vi "Test JSON Config.vi"() -> ()   [LabVIEW 2021]
uses:
  Source/Abs_Types/Double Float/Support/Type.ctl
  Source/Abs_Types/Boolean_1D/Support/Element Type.ctl
  Source/Constants/Support/DBL_1D/Type.ctl
  Source/Abs_Types/Double Float 1D/Support/Type.ctl
  Source/Abs_Types/Boolean/Abs_Boolean.lvclass
  C:/New folder/LV_Abstract/LV_Abstract/Source/Abs_Types/Type/Abs_Type.lvclass
  Source/Constants/Support/Bool_1D/Const_Bool_1D.lvclass
  Source/Abs_Types/Boolean_1D/Abs_Boolean_1D.lvclass
  Source/Constants/Support/DBL_1D/Const_DBL_1D.lvclass
  Source/Abs_Types/Type/Abs_Type.lvclass
  Source/Abs_Types/Double Float 1D/Abs_Double Float 1D.lvclass
  Source/Constants/Support/Bool_1D/Const_Bool_1D.lvclass/Const_Bool_1D.ctl
  Source/Constants/Support/DBL_1D/Const_DBL_1D.lvclass/Const_DBL_1D.ctl
  Source/Abs_Types/Type/Abs_Type.lvclass/Abs_Type.ctl
  Source/Abs_Types/Double Float/Abs_Double Float.lvclass
  Source/Abs_Types/String/Abs_String.lvclass
  Source/Abs_Types/String/Simple Read.vi
  Source/Abs_Types/Boolean/Simple Read.vi
  Source/Abs_Types/Double Float/Simple Read.vi
  Source/Constants/Support/DBL_1D/Properties/Write Value.vi
  Source/Constants/Support/Bool_1D/Properties/Write Value.vi
  Source/Abs_Types/Type/Properties/Write Name.vi
  Source/Abs_Types/Type/Properties/Read Name.vi
  Source/Constants/Support/Bool/Bool.vi
  Source/Functions/Logic/Support/OR/Bool/Method.vi
  Source/Constants/Support/DBL/DBL.vi
  Source/Constants/Support/Str/Str.vi
  Source/Constants/Support/DBL/Const_DBL.lvclass
  Source/Constants/Support/Bool/Const_Bool.lvclass
  Source/Functions/Logic/Support/OR/Bool/OR_Bool.lvclass
  Source/Constants/Support/Str/Const_Str.lvclass
panel:
  out "Value 3":T1
  out "JSON 6":string
  in  "Value 2":T2
  out "Boolean 1D":T3[](array[typedef])
  out "JSON":string
  in  "Array Value":bool[](array[boolean])
  out "Name":string
  out "JSON 5":string
  out "Boolean 6":bool
  in  "Boolean 5":bool
  in  "Boolean 4":bool
  out "String 2":string
  out "JSON 4":string
  in  "String":string
  out "Value":T4
  out "JSON 3":string
  in  "Numeric":dbl
  in  "Boolean 2":bool
  out "Boolean":bool
  out "JSON 2":string
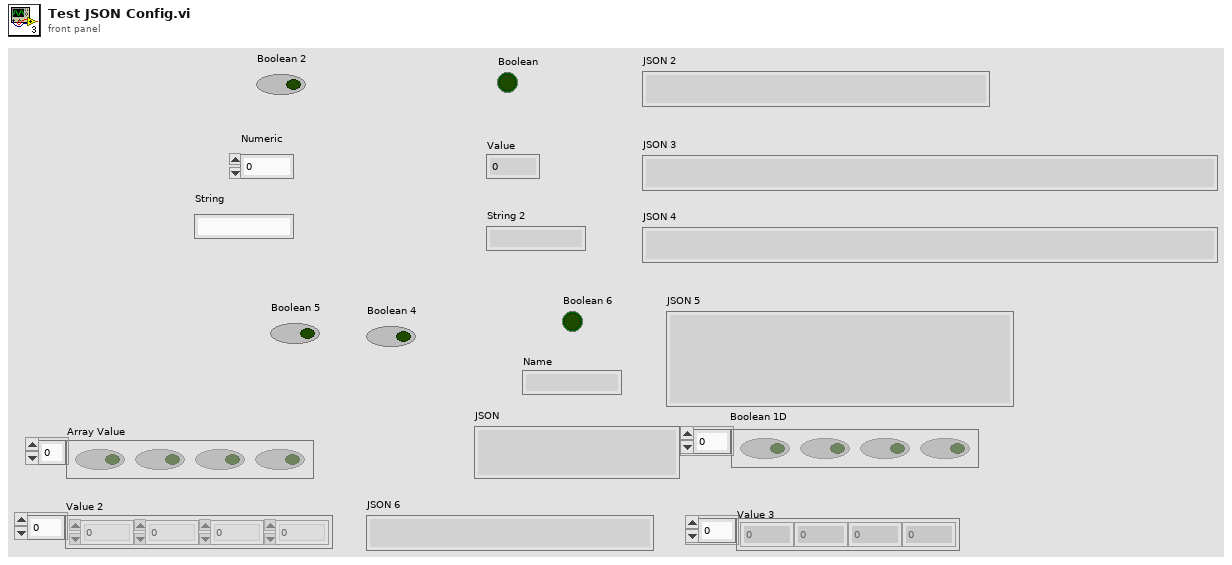
[diagram p1: front panel]
types:
  T1 = typedef "Abs_Double Float 1D.lvclass/Type.ctl" = dbl[]
  T2 = typedef "Const_DBL_1D.lvclass/Type.ctl" = dbl[]
  T3 = typedef "Abs_Boolean_1D.lvclass/Element Type.ctl" = bool
  T4 = typedef "Abs_Double Float.lvclass/Type.ctl" = dbl
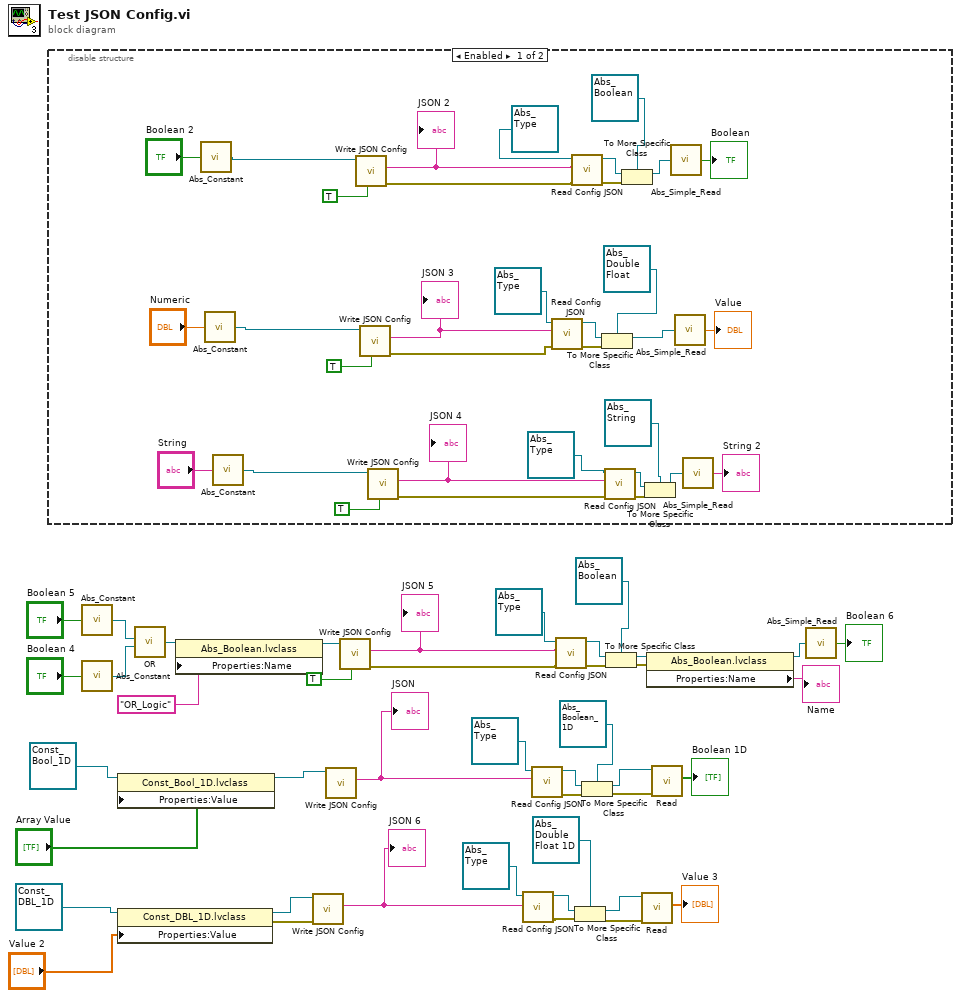
[diagram p0: block diagram]
diagram:
  n1 = disable-structure shown="Enabled" {
    frame Enabled {
      n2 = call-poly "Abs_Constant.vi"("Boolean"="Boolean 2") -> ("Abs_Boolean.lvclass"=w43:refnum<class "Abs_Boolean.lvclass">)  [unwired: 4 in]
      n3 = call-poly "Abs_Constant.vi"("Value"="Numeric") -> ("Constant"=w74:refnum<class "Const_DBL.lvclass">)  [unwired: 4 in]
      n4 = call-poly "Abs_Constant.vi"("String"="String") -> ("Abs_String.lvclass"=w53:refnum<class "Abs_String.lvclass">)  [unwired: 4 in]
      n5 = call-dynamic "Write JSON Config.vi"("Pretty Print?"=TRUE, "Abs_Type in"=w43) -> ("error out"=w60:errorcluster, "JSON"=w59:string)  [unwired: 7 in, 1 out]
      "JSON 2" <- w59
      n6 = call-dynamic "Write JSON Config.vi"("Pretty Print?"=TRUE, "Const_DBL in"=w74) -> ("error out"=w68:errorcluster, "JSON"=w65:string)  [unwired: 7 in, 1 out]
      "JSON 3" <- w65
      n7 = call-dynamic "Write JSON Config.vi"("Pretty Print?"=TRUE, "Abs_Type in"=w53) -> ("error out"=w46:errorcluster, "JSON"=w45:string)  [unwired: 7 in, 1 out]
      "JSON 4" <- w45
      n8 = call "Read Config JSON.vi"("error in (no error)"=w68, "JSON Config"=w65, "Abs_Type in"=refnum<class "Abs_Type.lvclass"> refnum) -> ("error out"=w70:errorcluster, "Abs_Type out"=w71:refnum<class "Abs_Type.lvclass">)  [unwired: 7 in]
      n9 = call "Read Config JSON.vi"("error in (no error)"=w60, "JSON Config"=w59, "Abs_Type in"=refnum<class "Abs_Type.lvclass"> refnum) -> ("error out"=w58:errorcluster, "Abs_Type out"=w57:refnum<class "Abs_Type.lvclass">)  [unwired: 7 in]
      n10 = To More Specific Class(target class=refnum<class "Abs_Double Float.lvclass"> refnum ("Class"), reference=w71, error in=w70) -> (specific class reference=w67:refnum<class "Abs_Double Float.lvclass">)  [unwired: 1 out]
      n11 = call "Read Config JSON.vi"("error in (no error)"=w46, "JSON Config"=w45, "Abs_Type in"=refnum<class "Abs_Type.lvclass"> refnum) -> ("error out"=w48:errorcluster, "Abs_Type out"=w44:refnum<class "Abs_Type.lvclass">)  [unwired: 7 in]
      n12 = To More Specific Class(target class=refnum<class "Abs_Boolean.lvclass"> refnum ("Boolean in"), reference=w57, error in=w58) -> (specific class reference=w55:refnum<class "Abs_Boolean.lvclass">)  [unwired: 1 out]
      n13 = To More Specific Class(target class=refnum<class "Abs_String.lvclass"> refnum ("Abs_String in"), reference=w44, error in=w48) -> (specific class reference=w49:refnum<class "Abs_String.lvclass">)  [unwired: 1 out]
      n14 = call-poly "Abs_Simple_Read.vi"("Boolean in"=w55) -> ("Boolean"=→"Boolean":bool)  [unwired: 4 in]
      n15 = call-poly "Abs_Simple_Read.vi"("Class"=w67) -> ("Value"=→"Value":dbl)  [unwired: 4 in]
      n16 = call-poly "Abs_Simple_Read.vi"("Abs_String in"=w49) -> ("String"=→"String 2":string)  [unwired: 4 in]
    }
    frame Disabled {
    }
  }
  n17 = call-poly "Abs_Constant.vi"("Boolean"="Boolean 5") -> ("Abs_Boolean.lvclass"=w32:refnum<class "Abs_Boolean.lvclass">)  [unwired: 4 in]
  n18 = call-poly "Abs_Constant.vi"("Boolean"="Boolean 4") -> ("Abs_Boolean.lvclass"=w31:refnum<class "Abs_Boolean.lvclass">)  [unwired: 4 in]
  n19 = property class="Const_Bool_1D.lvclass"(reference=refnum<class "Const_Bool_1D.lvclass"> refnum ("Const_Bool_1D.lvclass"), "Properties:Value"="Array Value") -> (reference out=w21:refnum<class "Const_Bool_1D.lvclass">)  [unwired: 1 in, 1 out]
  n20 = property class="Const_DBL_1D.lvclass"(reference=refnum<class "Const_DBL_1D.lvclass"> refnum ("Const_DBL_1D.lvclass"), "Properties:Value"="Value 2") -> (reference out=w10:refnum<class "Const_DBL_1D.lvclass">, error out=w1:errorcluster)  [unwired: 1 in]
  n21 = call-poly "OR.vi"("B"=w31, "A"=w32) -> ("Result"=w30:refnum<class "Abs_Boolean.lvclass">)  [unwired: 4 in]
  n22 = property class="Abs_Boolean.lvclass"(reference=w30, "Properties:Name"="OR_Logic" ("Name")) -> (reference out=w29:refnum<class "Abs_Boolean.lvclass">)  [unwired: 1 in, 1 out]
  n23 = call-dynamic "Write JSON Config.vi"("error in (no error)"=w1, "Const_DBL in"=w10) -> ("JSON"=w8:string)  [unwired: 7 in, 2 out]
  "JSON 6" <- w8
  n24 = call-dynamic "Write JSON Config.vi"("Const_Bool in"=w21) -> ("JSON"=w17:string)  [unwired: 8 in, 2 out]
  "JSON" <- w17
  n25 = call-dynamic "Write JSON Config.vi"("Pretty Print?"=TRUE, "Abs_Type in"=w29) -> ("error out"=w37:errorcluster, "JSON"=w38:string)  [unwired: 7 in, 1 out]
  "JSON 5" <- w38
  n26 = call "Read Config JSON.vi"("JSON Config"=w8, "Abs_Type in"=refnum<class "Abs_Type.lvclass"> refnum) -> ("error out"=w7:errorcluster, "Abs_Type out"=w6:refnum<class "Abs_Type.lvclass">)  [unwired: 8 in]
  n27 = call "Read Config JSON.vi"("JSON Config"=w17, "Abs_Type in"=refnum<class "Abs_Type.lvclass"> refnum) -> ("error out"=w20:errorcluster, "Abs_Type out"=w19:refnum<class "Abs_Type.lvclass">)  [unwired: 8 in]
  n28 = call "Read Config JSON.vi"("error in (no error)"=w37, "JSON Config"=w38, "Abs_Type in"=refnum<class "Abs_Type.lvclass"> refnum) -> ("error out"=w39:errorcluster, "Abs_Type out"=w40:refnum<class "Abs_Type.lvclass">)  [unwired: 7 in]
  n29 = To More Specific Class(target class=refnum<class "Abs_Double Float 1D.lvclass"> refnum ("Abs_Double Float 1D.lvclass"), reference=w6, error in=w7) -> (specific class reference=w4:refnum<class "Abs_Double Float 1D.lvclass">, error out=w3:errorcluster)
  n30 = To More Specific Class(target class=refnum<class "Abs_Boolean_1D.lvclass"> refnum ("Abs_Boolean_1D.lvclass"), reference=w19, error in=w20) -> (specific class reference=w15:refnum<class "Abs_Boolean_1D.lvclass">, error out=w14:errorcluster)
  n31 = To More Specific Class(target class=refnum<class "Abs_Boolean.lvclass"> refnum ("Boolean in"), reference=w40, error in=w39) -> (specific class reference=w26:refnum<class "Abs_Boolean.lvclass">, error out=w27:errorcluster)
  n32 = call-dynamic "Read.vi"("error in (no error)"=w3, "Double Float.lvclass_340760 in"=w4) -> ("Value"=→"Value 3":T1)  [unwired: 7 in, 2 out]
  n33 = property class="Abs_Boolean.lvclass"(reference=w26, error in=w27) -> (reference out=w25:refnum<class "Abs_Boolean.lvclass">, "Properties:Name"=→"Name":string)  [unwired: 1 out]
  n34 = call-dynamic "Read.vi"("error in (no error)"=w14, "Boolean in"=w15) -> ("Boolean 1D"=→"Boolean 1D":T3[])  [unwired: 7 in, 2 out]
  n35 = call-poly "Abs_Simple_Read.vi"("Boolean in"=w25) -> ("Boolean"=→"Boolean 6":bool)  [unwired: 4 in]
